vi "Read XML HW Configuration File_Extra Checks_Check Tx Label Rates For Each hardWareChannel.vi"(8 "error in (no error)":errorcluster, 11 "Array In":T1[](array[typedef]) {"speed" items=["Auto", "Low", "High"]; "Labels"."scheduleBuildUnit" items=["Millisecond", "Microsecond"]}) -> (0 "error out":errorcluster)   [LabVIEW 2020]
doc: "This VI checks that for a given Hardware Channel, each Label Name is unique."
uses:
  Controls/Ballard_Channel.ctl
  Controls/Ballard_Label.ctl
  Controls/Ballard_Word.ctl
  Controls/ARINCParam.ctl
  Shared/Controls and Global/TransferType.ctl
  Controls/Channel_direction.ctl
  Controls/Channel Speed.ctl
  Shared/Ballard Arinc-429 Shared.lvlib
  Ballard Arinc-429 System Explorer.lvlib
panel:
  out "Error Source":string
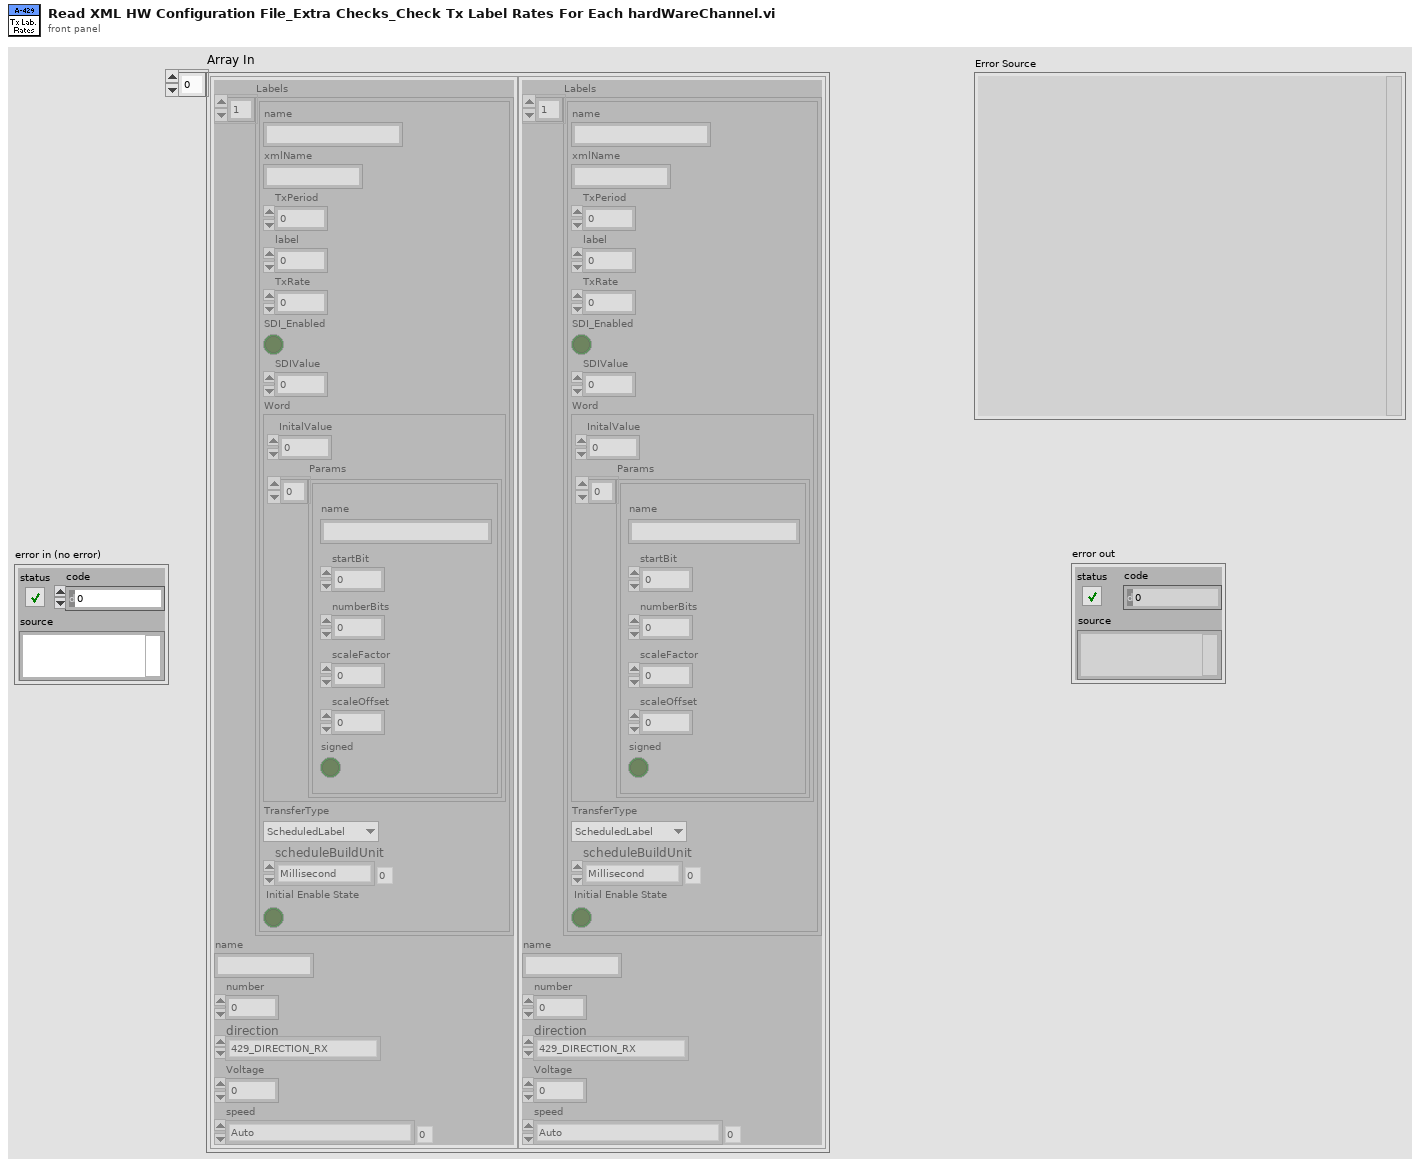
[diagram p1: front panel]
types:
  T1 = typedef "Ballard Arinc-429 System Explorer.lvlib/Ballard_Channel.ctl" = cluster{"Labels":T2[], "name":string, "number":u8, "direction":T6, "Voltage":dbl, "speed":T7}
  T2 = typedef "Ballard Arinc-429 System Explorer.lvlib/Ballard_Label.ctl" = cluster{"name":string, "xmlName":string, "TxPeriod":u32, "label":u32, "TxRate":dbl, "SDI_Enabled":bool, "SDIValue":u8, "Word":T3, "TransferType":T5, "scheduleBuildUnit":i32, "Initial Enable State":bool}
  T3 = typedef "Ballard Arinc-429 System Explorer.lvlib/Ballard_Word.ctl" = cluster{"InitalValue":u32, "Params":T4[]}
  T4 = typedef "Ballard Arinc-429 System Explorer.lvlib/ARINCParam.ctl" = cluster{"name":string, "startBit":i32, "numberBits":i32, "scaleFactor":dbl, "scaleOffset":dbl, "signed":bool}
  T5 = typedef "Ballard Arinc-429 Shared.lvlib/TransferType.ctl" = enum16{"ScheduledLabel", "Acyclic", "Block", "Strobe"}
  T6 = typedef "Ballard Arinc-429 System Explorer.lvlib/Channel_direction.ctl" = enum16{"429_DIRECTION_RX", "429_DIRECTION_TX"}
  T7 = typedef "Ballard Arinc-429 System Explorer.lvlib/Channel Speed.ctl" = i32
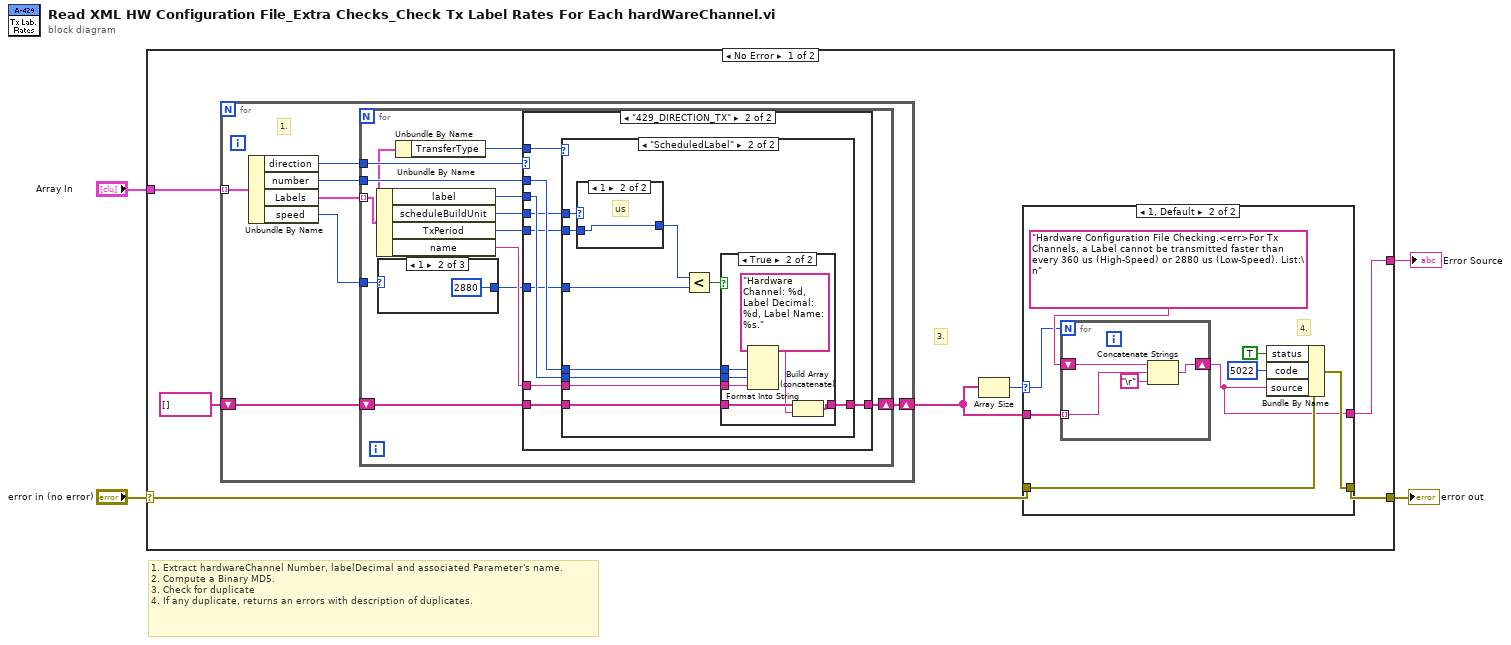
[diagram p0: block diagram]
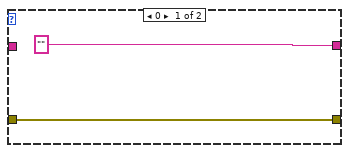
[diagram p2: hidden frame]
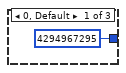
[diagram p3: hidden frame]
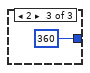
[diagram p4: hidden frame]
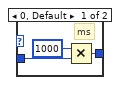
[diagram p8: hidden frame]
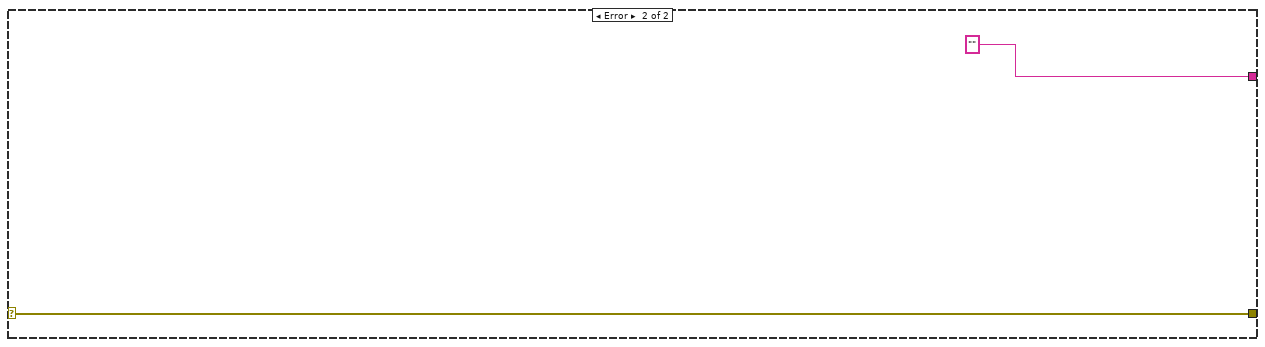
[diagram p9: hidden frame]
diagram:
  # "1. Extract hardwareChannel Number, labelDecimal and associated Parameter's name.\n2. Compute a Binary MD5.\n3. Check for duplicate\n4. If any duplicate, returns an errors with description of duplicates."
  n1 = case shown="No Error" "error in (no error)" {
    selector: "error in (no error)" -> [w10 w82]
    tunnel: [w8 w82] -> w3
    tunnel: "Array In" -> [w9 _]
    tunnel: [w7 ""] -> w1
    frame No Error {
      # "3."
      n2 = for {
        tunnel: w9 -> [w32] mode=indexing
        shift-right: [w28] -> w5
        shift-left: string[] [] -> [w29]
        # "1."
        n3 = Unbundle By Name(w32) -> ("direction"=w26:T6, "number"=w31:u8, "Labels"=w30:T2[], "speed"=w27:T7)
        n4 = for {
          tunnel: w31 -> [w40]
          tunnel: w30 -> [w34] mode=indexing
          shift-right: [w42] -> w28
          shift-left: w29 -> [w43]
          tunnel: w27 -> [w37]
          tunnel: w26 -> [w35]
          n5 = Unbundle By Name(w34) -> ("label"=w44:u32, "scheduleBuildUnit"=w39:i32, "TxPeriod"=w38:u32, "name"=w41:string)
          n6 = case shown="1" w37 {
            tunnel: [u32 4294967295 u32 2880 u32 360] -> w36
            frame 0, Default {
            }
            frame 1 {
            }
            frame 2 {
            }
          }
          n7 = Unbundle By Name(w34) -> ("TransferType"=w33:T5)
          n8 = case shown="\"429_DIRECTION_TX\"" w35 {
            tunnel: w44 -> [_ w57]
            tunnel: w43 -> [w48 w56]
            tunnel: [w48 w55] -> w42
            tunnel: w41 -> [_ w54]
            tunnel: w40 -> [_ w53]
            tunnel: w39 -> [_ w52]
            tunnel: w38 -> [_ w51]
            tunnel: w36 -> [_ w50]
            tunnel: w33 -> [_ w49]
            frame "429_DIRECTION_RX", Default {
              # "It's a Rx Channel"
            }
            frame "429_DIRECTION_TX" {
              n9 = case shown="\"ScheduledLabel\"" w49 {
                tunnel: w57 -> [_ w68]
                tunnel: w56 -> [w58 w67]
                tunnel: [w58 w66] -> w55
                tunnel: w54 -> [_ w65]
                tunnel: w53 -> [_ w64]
                tunnel: w52 -> [_ w63]
                tunnel: w51 -> [_ w62]
                tunnel: w50 -> [_ w60]
                frame Default {
                }
                frame "ScheduledLabel" {
                  n10 = case shown="1" w63 {
                    tunnel: w62 -> [w79 w80]
                    tunnel: [w77 w80] -> w61
                    frame 0, Default {
                      # "ms"
                      n11 = Multiply(x=u32 1000, y=w79) -> (x*y=w77:u32)
                    }
                    frame 1 {
                      # "us"
                    }
                  }
                  n12 = Less?(x=w61, y=w60) -> (x < y?=w59:bool)
                  n13 = case shown="True" w59 {
                    tunnel: w68 -> [_ w76]
                    tunnel: w67 -> [w69 w75]
                    tunnel: [w69 w74] -> w66
                    tunnel: w65 -> [_ w71]
                    tunnel: w64 -> [_ w70]
                    frame False {
                    }
                    frame True {
                      n14 = Format Into String(format string="Hardware Channel: %d, Label Decimal: %d, Label Name: %s.", w70, w76, w71) -> (resulting string=w72:string)  [unwired: 2 in, 1 out]
                      n15 = Build Array (concatenate)(w75, w72) -> (w74:string[])
                    }
                  }
                }
              }
            }
          }
        }
      }
      n16 = Array Size(array=w5) -> (size(s)=w11:i32)
      n17 = case shown="1, Default" w11 {
        selector: w11 -> [_ w16]
        tunnel: w10 -> [w13 w21]
        tunnel: w5 -> [_ w15]
        tunnel: [w13 w20] -> w8
        tunnel: ["" w14] -> w7
        frame 0 {
        }
        frame 1, Default {
          # "4."
          n18 = for {
            N: w16 -> [_]
            shift-right: [w24] -> w14
            shift-left: "Hardware Configuration File Checking.<err>For Tx Channels, a Label cannot be transmitted faster than every 360 us (High-Speed) or 2880 us (Low-Speed). List:\n" -> [w25]
            tunnel: w15 -> [w22] mode=indexing
            n19 = Concatenate Strings(w25, w22, "\r") -> (w24:string)
          }
          n20 = Bundle By Name(cluster=w21, "status"=TRUE, "code"=5022, "source"=w14) -> (w20:errorcluster)
        }
      }
    }
    frame Error {
    }
  }
  "error out" <- w3
  "Error Source" <- w1
